vi "主VI.vi"() -> ()   [LabVIEW 2011]
panel:
  out "Array 2":i32[](array[numeric])
  out "Array":i32[](array[numeric])
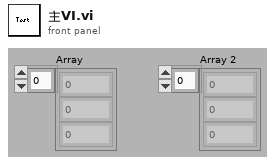
[diagram p1: front panel]
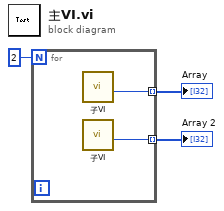
[diagram p0: block diagram]
diagram:
  n1 = for {
    N: 2 -> [_]
    tunnel: [w5] -> w2 mode=indexing
    tunnel: [w4] -> w1 mode=indexing
    n2 = call "子VI.vi"() -> ("output"=w5:i32)  [unwired: 11 in]
    n3 = call "子VI.vi"() -> ("output"=w4:i32)  [unwired: 11 in]
  }
  "Array" <- w2
  "Array 2" <- w1
